vi "Visualise found peak.vi"(8 "error in (no error)":errorcluster, 10 "Found Peak":refnum<data-value>, 11 "UI Root in":refnum<class "UI Root.lvclass">) -> (0 "error out":errorcluster, 3 "UI Root out":refnum<class "UI Root.lvclass">)   [LabVIEW 2020, in "UI Root.lvlib" / "UI Root.lvclass"]
uses:
  UI Root.lvclass
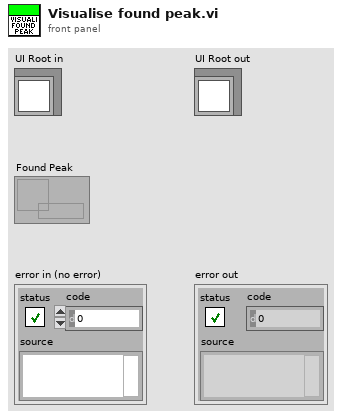
[diagram p1: front panel]
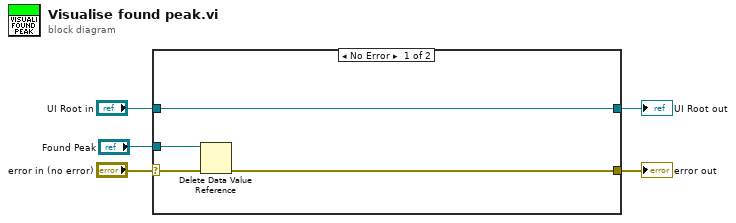
[diagram p0: block diagram]
diagram:
  n1 = case shown="No Error" "error in (no error)" {
    selector: "error in (no error)" -> [w7 w11]
    tunnel: [w6 w11] -> w4
    tunnel: [w9 w10] -> w2
    tunnel: "UI Root in" -> [w9 w10]
    tunnel: "Found Peak" -> [w8 _]
    frame No Error {
      n2 = Delete Data Value Reference(data value reference=w8, error in=w7) -> (error out=w6:errorcluster)  [unwired: 1 out]
    }
    frame Error {
    }
  }
  "error out" <- w4
  "UI Root out" <- w2
